vi "ABB enter winding data.vi"(9 "Efficiency Units":u16(ring) items=["METRIC", "IMPERIAL", "", "", ""], 10 "Efficiency Standard":u16(ring) items=["IEC", "NEMA"], 11 "Motor Type":u16(ring) items=["Wound Induction Motor", "Induction Motor", "Synchronous Motor", "Synchronous Generator"]) -> (3 "entered data":string[][](array[string]))   [LabVIEW 2017]
uses:
  <vilib>/Analysis/baseanly.llb/Mean (DBL).vi
  ABB global.vi
  <vilib>/Analysis/NI_AALBase.lvlib
panel:
  in  "Wound Motor Voltage Ratio":T1
  out "Winding ºC":T2 {"Avrg ºC" format="%#.3g"; "Temperature (ºC)" format="%#.2g"}
  out "Additional Temp":T3 {"Avrg cold air ºC" format="%#.3g"; "Avrg warm air ºC" format="%#.3g"; "Cold Air  (ºC)" format="%#.2g"; "Warm Air  (ºC)" format="%#.2g"}
  in  "Additional RTDs":T4={"Warm Air Ohms"=[], "Cold Air Ohms"=[], "No. Warm Air"=4, "No. Cold Air"=6} {"No. Cold Air" min=0 max=12; "No. Warm Air" min=0 max=6}
  in  "Rotor Winding Resistance":T5 {"Units" items=["Ohms", "mOhms", "uOhms"]; "Rotor K - M" format="%#.6g"; "Rotor L - M" format="%#.6g"; "Rotor K -L" format="%#.6g"}
  in  "Stator Winding resistance":T6 {"Stator U - W" format="%#.6g"; "Stator V - W" format="%#.6g"; "Units" items=["Ohms", "mOhms", "uOhms"]; "Stator U - V" format="%#.6g"}
  in  "Winding Temperatures":T7={"No. Winding ETDs"=6, "Detector Ohms"=[]} {"No. Winding ETDs" min=1 max=12}
  in  "Exit":bool
  # "Enter Winding data"
  # "20%"
  # "100%"
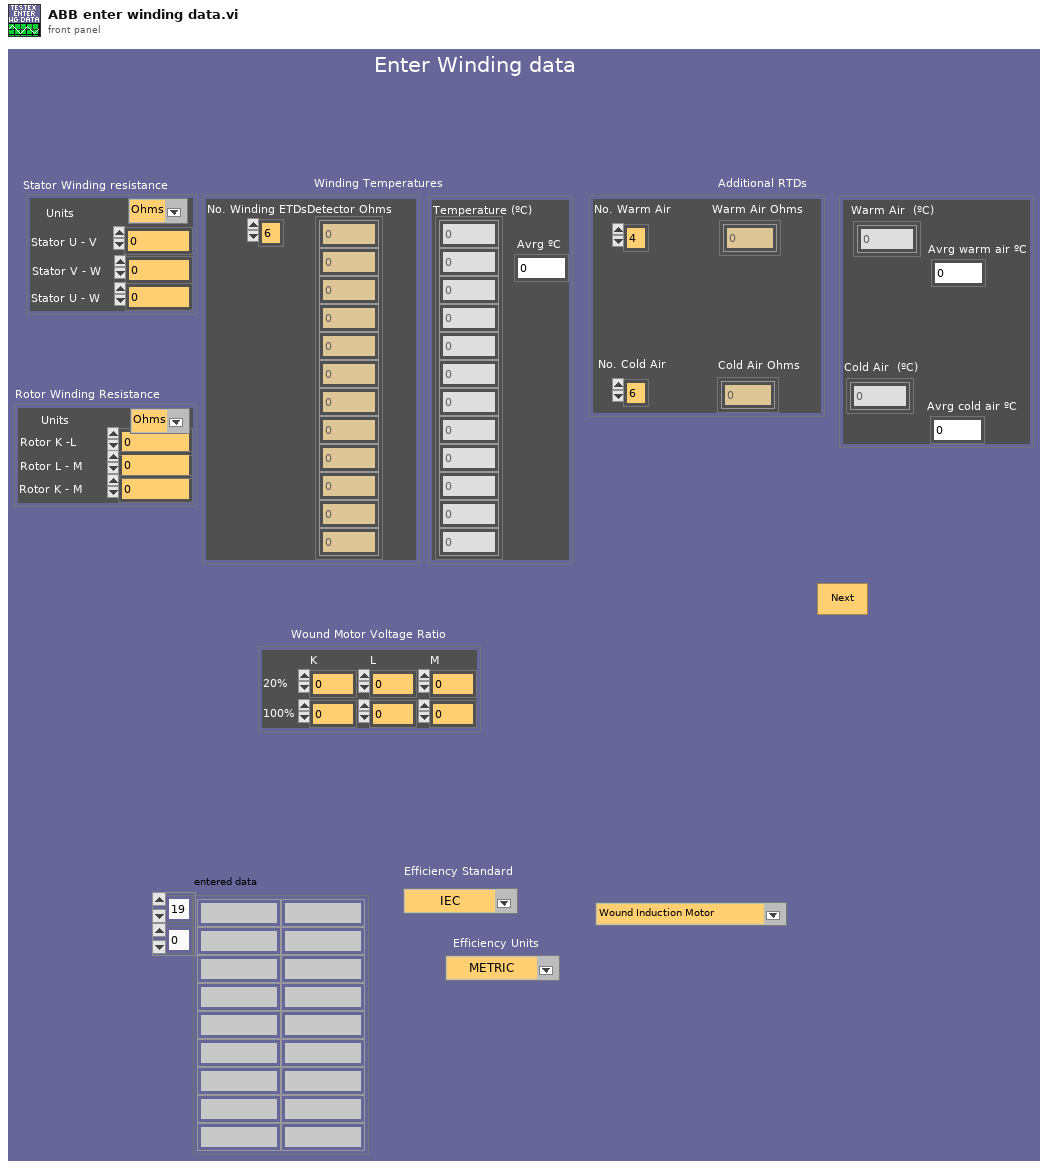
[diagram p1: front panel]
types:
  T1 = cluster{"K-20":dbl, "L-20":dbl, "M-20":dbl, "K-100":dbl, "L-100":dbl, "M-100":dbl}
  T2 = cluster{"Temperature (ºC) ":dbl[], "Avrg ºC ":dbl}
  T3 = cluster{"Warm Air  (ºC) ":dbl[], "Cold Air  (ºC) ":dbl[], "Avrg warm air ºC ":dbl, "Avrg cold air ºC":dbl}
  T4 = cluster{"Warm Air Ohms":dbl[], "Cold Air Ohms":dbl[], "No. Warm Air":i32, "No. Cold Air":i32}
  T5 = cluster{"Units":u16, "Rotor K -L":dbl, "Rotor L - M ":dbl, "Rotor K - M":dbl}
  T6 = cluster{"Units":u16, "Stator U - V":dbl, "Stator V - W":dbl, "Stator U - W":dbl}
  T7 = cluster{"No. Winding ETDs":i32, "Detector Ohms":dbl[]}
  T8 = cluster{"Selected Entries[0]":string, "Selected Entries[1]":string, "Selected Entries[2]":string, "Selected Entries[3]":string}
  T9 = cluster{"Selected Entries[0]":string, "Selected Entries[1]":string, "Selected Entries[2]":string, "Selected Entries[3]":string, "Selected Entries[4]":string}
  T10 = cluster{"Selected Entries[0]":dbl, "Selected Entries[1]":dbl, "Selected Entries[2]":dbl, "Selected Entries[3]":dbl}
  T11 = cluster{"Selected Entries[0]":dbl, "Selected Entries[1]":dbl, "Selected Entries[2]":dbl, "Selected Entries[3]":dbl, "Selected Entries[4]":dbl}
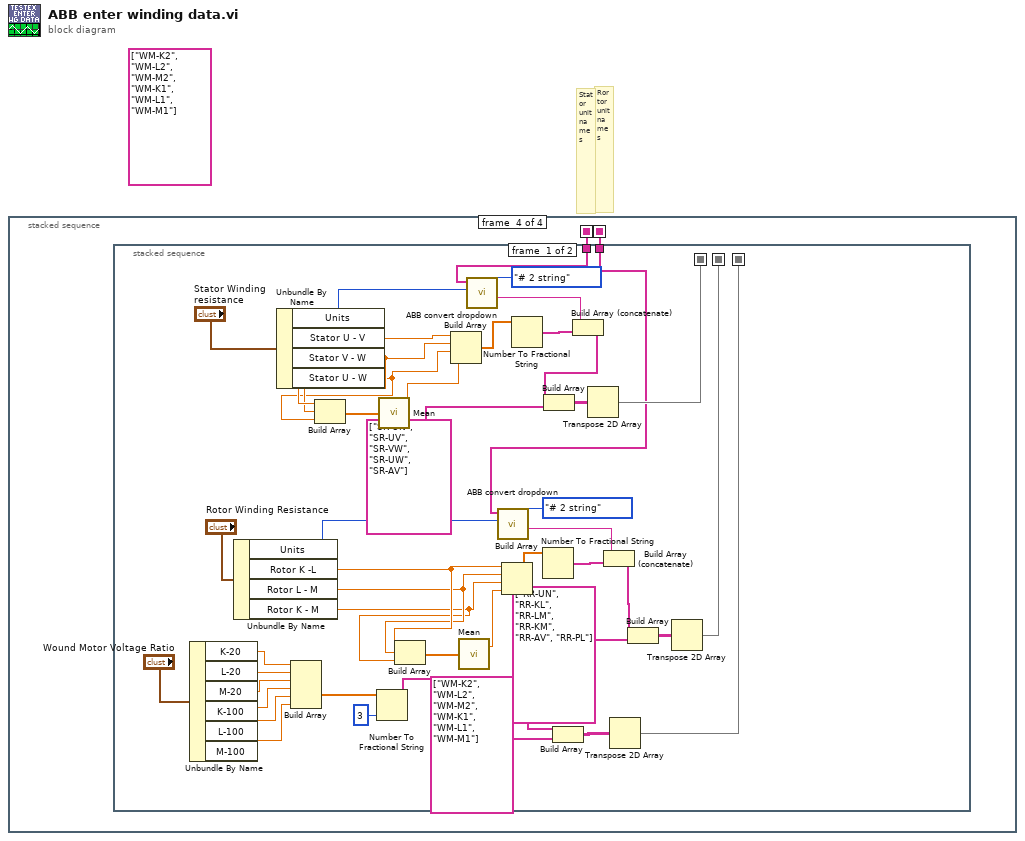
[diagram p0: block diagram]
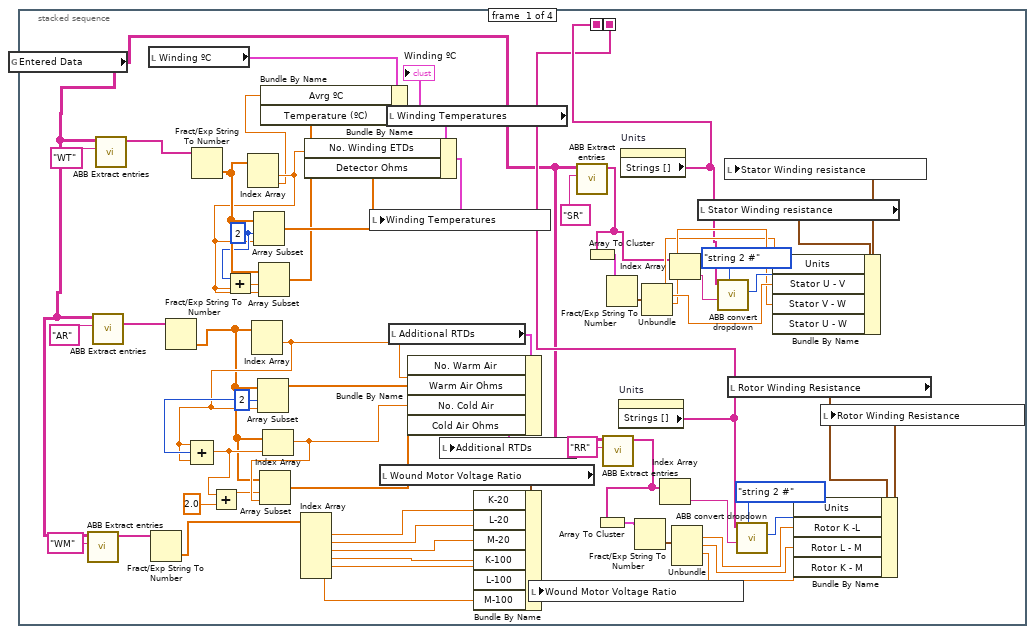
[diagram p2: hidden frame]
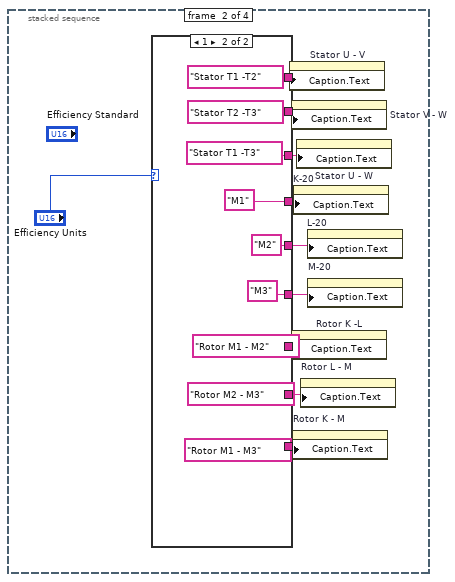
[diagram p3: hidden frame]
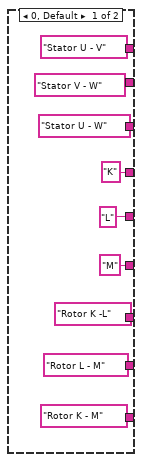
[diagram p4: hidden frame]
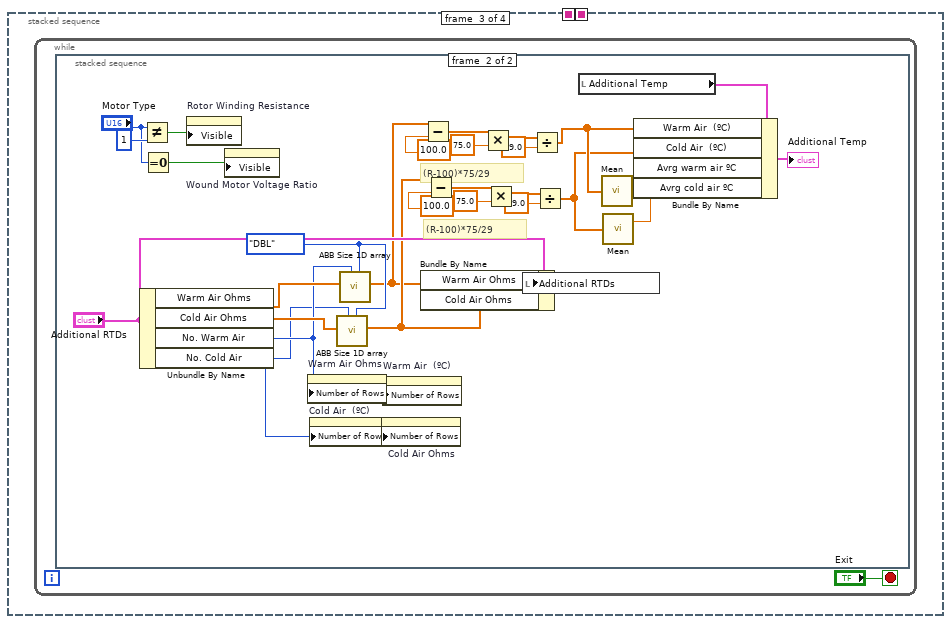
[diagram p5: hidden frame]
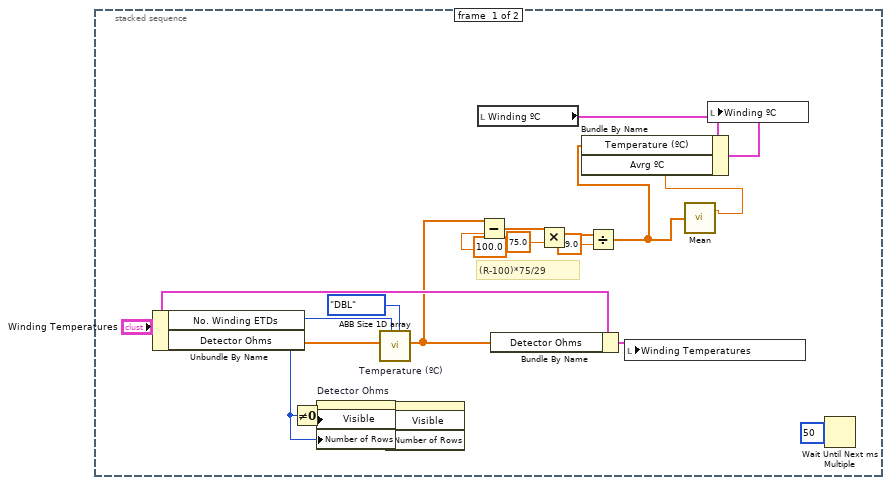
[diagram p6: hidden frame]
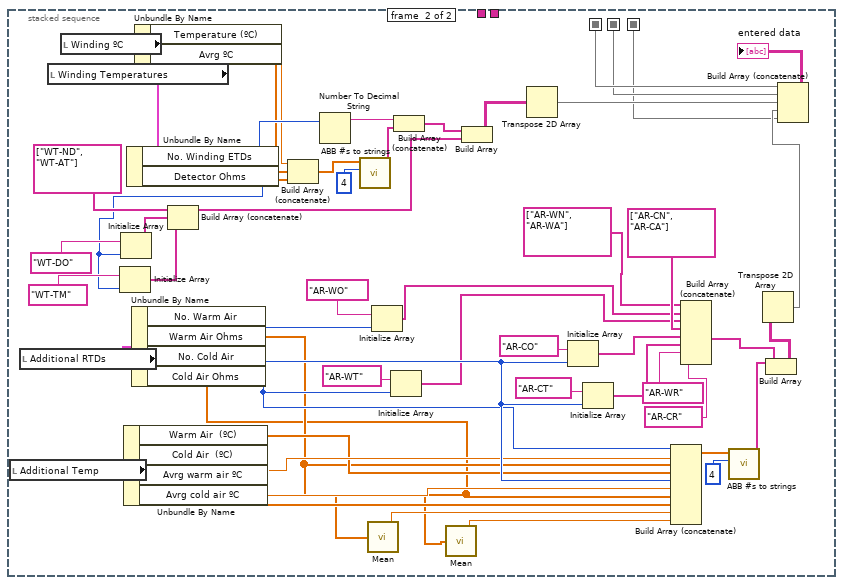
[diagram p7: hidden frame]
diagram:
  (unwired) string[] ["WM-K2", "WM-L2", "WM-M2", "WM-K1", "WM-L1", "WM-M1"]
  # "Rortor unit names"
  # "Stator unit names"
  n1 = stacked-sequence {
    seq-local: [w36 _ _ _] -> [_ _ _ w141]
    seq-local: [w35 _ _ _] -> [_ _ _ w140]
    frame #0 {
      w25 = 2 ("index")
      w32 = 2 ("index")
      n2 = global read "ABB global.vi" "Entered Data"() -> (w12:string[][])
      n3 = call "ABB Extract entries.vi"("Entry ID"="WM", "Entry table in"=w12) -> ("Selected Entries"=w10:string[])  [unwired: 9 in]
      n4 = call "ABB Extract entries.vi"("Entry ID"="AR", "Entry table in"=w12) -> ("Selected Entries"=w28:string[])  [unwired: 9 in]
      n5 = call "ABB Extract entries.vi"("Entry ID"="WT", "Entry table in"=w12) -> ("Selected Entries"=w60:string[])  [unwired: 9 in]
      n6 = local read "Winding ºC"() -> (w18:T2)
      n7 = Fract/Exp String To Number(string=w10) -> (number=w9:dbl[])  [unwired: 3 in, 1 out]
      n8 = Fract/Exp String To Number(string=w28) -> (number=w14:dbl[])  [unwired: 3 in, 1 out]
      n9 = Fract/Exp String To Number(string=w60) -> (number=w33:dbl[])  [unwired: 3 in, 1 out]
      n10 = Index Array(array=w33) -> (element #1=w31:dbl, element #2=w16:dbl)  [unwired: 2 in]
      n11 = Add(x=w32, y=w31) -> (x+y=w30:dbl)
      n12 = Index Array(array=w14) -> (element #1=w24:dbl)  [unwired: 2 in, 1 out]
      n13 = Compound Arithmetic op=ADD(w24, w25, w24) -> (w23:dbl)
      n14 = Add(x=w23, y=2.0) -> (x+y=w13:dbl)
      n15 = Array Subset(array=w33, index=w32, length=w31) -> (w62:dbl[])
      n16 = Array Subset(array=w14, index=w25, length=w24) -> (w26:dbl[])
      n17 = Array Subset(array=w33, index=w30, length=w31) -> (w15:dbl[])
      n18 = Bundle By Name(cluster=w18, "Avrg ºC"=w16, "Temperature (ºC)"=w15) -> (→"Winding ºC":T2)
      n19 = Index Array(array=w14, index=w23) -> (element=w21:dbl)
      n20 = Array Subset(array=w14, index=w13, length=w21) -> (w20:dbl[])
      n21 = Index Array(array=w9) -> (element #1=w7:dbl, element #2=w6:dbl, element #3=w5:dbl, element #4=w4:dbl, element #5=w3:dbl, element #6=w2:dbl)  [unwired: 6 in]
      n22 = local read "Wound Motor Voltage Ratio"() -> (w8:T1)
      n23 = local read "Winding Temperatures"() -> (w64:T7)
      n24 = Bundle By Name(cluster=w64, "No. Winding ETDs"=w31, "Detector Ohms"=w62) -> (w63:T7)
      n25 = local write "Winding Temperatures"(w63) -> ()
      n26 = local read "Additional RTDs"() -> (w27:T4)
      n27 = Bundle By Name(cluster=w27, "No. Warm Air"=w24, "Warm Air Ohms"=w26, "No. Cold Air"=w21, "Cold Air Ohms"=w20) -> (w19:T4)
      n28 = local write "Additional RTDs"(w19) -> ()
      n29 = Bundle By Name(cluster=w8, "K-20"=w7, "L-20"=w6, "M-20"=w5, "K-100"=w4, "L-100"=w3, "M-100"=w2) -> (w1:T1)
      n30 = local write "Wound Motor Voltage Ratio"(w1) -> ()
      n31 = call "ABB Extract entries.vi"("Entry ID"="SR", "Entry table in"=w12) -> ("Selected Entries"=w49:string[])  [unwired: 9 in]
      n32 = Array To Cluster(array=w49) -> (cluster=w50:T8)
      n33 = call "ABB Extract entries.vi"("Entry ID"="RR", "Entry table in"=w12) -> ("Selected Entries"=w38:string[])  [unwired: 9 in]
      n34 = Array To Cluster(array=w38) -> (cluster=w41:T9)
      n35 = Fract/Exp String To Number(string=w50) -> (number=w57:T10)  [unwired: 3 in, 1 out]
      n36 = property on="Units" class="Ring (strict)"() -> ("Strings []"=w35:string[])  [unwired: 2 in, 2 out]
      n37 = property on="Units" class="Ring (strict)"() -> ("Strings []"=w36:string[])  [unwired: 2 in, 2 out]
      n38 = Fract/Exp String To Number(string=w41) -> (number=w42:T11)  [unwired: 3 in, 1 out]
      n39 = Unbundle(w57) -> ("Selected Entries[1]"=w54:dbl, "Selected Entries[2]"=w53:dbl, "Selected Entries[3]"=w52:dbl)  [unwired: 1 out]
      n40 = Index Array(array=w38) -> (element=w37:string)  [unwired: 1 in]
      n41 = Index Array(array=w49) -> (element=w48:string)  [unwired: 1 in]
      n42 = Unbundle(w42) -> ("Selected Entries[1]"=w45:dbl, "Selected Entries[2]"=w46:dbl, "Selected Entries[3]"=w47:dbl)  [unwired: 2 out]
      n43 = local read "Stator Winding resistance"() -> (w59:T6)
      n44 = call "ABB convert dropdown.vi"("Mode"=enum16{"# 2 string", "string 2 #"}."string 2 #", "String in"=w48, "Strings"=w36) -> ("#out"=w56:i32)  [unwired: 7 in, 1 out]
      n45 = local read "Rotor Winding Resistance"() -> (w40:T5)
      n46 = call "ABB convert dropdown.vi"("Mode"=enum16{"# 2 string", "string 2 #"}."string 2 #", "String in"=w37, "Strings"=w35) -> ("#out"=w43:i32)  [unwired: 7 in, 1 out]
      n47 = Bundle By Name(cluster=w59, "Units"=w56, "Stator U - V"=w54, "Stator V - W"=w53, "Stator U - W"=w52) -> (w58:T6)
      n48 = local write "Stator Winding resistance"(w58) -> ()
      n49 = Bundle By Name(cluster=w40, "Units"=w43, "Rotor K -L"=w45, "Rotor L - M"=w46, "Rotor K - M"=w47) -> (w39:T5)
      n50 = local write "Rotor Winding Resistance"(w39) -> ()
    }
    frame #1 {
      n51 = case shown="1" "Efficiency Units" {
        tunnel: ["Stator U - V" ("Caption.Text") "Stator T1 -T2" ("Caption.Text")] -> w74
        tunnel: ["Stator V - W" ("Caption.Text") "Stator T2 -T3" ("Caption.Text")] -> w73
        tunnel: ["Stator U - W" ("Caption.Text") "Stator T1 -T3" ("Caption.Text")] -> w72
        tunnel: ["K" ("Caption.Text") "M1" ("Caption.Text")] -> w69
        tunnel: ["L" ("Caption.Text") "M2" ("Caption.Text")] -> w71
        tunnel: ["M" ("Caption.Text") "M3" ("Caption.Text")] -> w70
        tunnel: ["Rotor K -L" "Rotor M1 - M2"] -> w68
        tunnel: ["Rotor L - M" "Rotor M2 - M3"] -> w67
        tunnel: ["Rotor K - M" "Rotor M1 - M3"] -> w66
        frame 0, Default {
        }
        frame 1 {
        }
      }
      n52 = property on="Stator U - V" class="DigNum (strict)"("Caption.Text"=w74) -> ()  [unwired: 2 in, 2 out]
      n53 = property on="Stator V - W" class="DigNum (strict)"("Caption.Text"=w73) -> ()  [unwired: 2 in, 2 out]
      n54 = property on="Rotor K -L" class="DigNum (strict)"("Caption.Text"=w68) -> ()  [unwired: 2 in, 2 out]
      n55 = property on="Rotor K - M" class="DigNum (strict)"("Caption.Text"=w66) -> ()  [unwired: 2 in, 2 out]
      n56 = property on="K-20" class="DigNum (strict)"("Caption.Text"=w69) -> ()  [unwired: 2 in, 2 out]
      n57 = property on="Stator U - W" class="DigNum (strict)"("Caption.Text"=w72) -> ()  [unwired: 2 in, 2 out]
      n58 = property on="Rotor L - M" class="DigNum (strict)"("Caption.Text"=w67) -> ()  [unwired: 2 in, 2 out]
      n59 = property on="L-20" class="DigNum (strict)"("Caption.Text"=w71) -> ()  [unwired: 2 in, 2 out]
      n60 = property on="M-20" class="DigNum (strict)"("Caption.Text"=w70) -> ()  [unwired: 2 in, 2 out]
    }
    frame #2 {
      n61 = while {
        stop <- "Exit" stop-if-true
        n62 = stacked-sequence {
          frame #0 {
            # "(R-100)*75/29"
            n63 = Unbundle By Name("Winding Temperatures") -> ("No. Winding ETDs"=w104:i32, "Detector Ohms"=w108:dbl[])
            n64 = Not Equal To 0?(x=w104) -> (x != 0?=w105:bool)
            n65 = property on="Detector Ohms" class="Arr (strict)"("Visible"=w105, "Number of Rows"=w104) -> ()  [unwired: 2 in, 2 out]
            n66 = call "ABB Size 1D array.vi"("Type"=enum16{"Integer", "DBL", "STRING", "BOOLEAN"}."DBL", "Size"=w104, "DBL Array In"=w108) -> ("DBL Array out"=w99:dbl[])  [unwired: 5 in, 3 out]
            n67 = property on="Temperature (ºC)" class="Arr (strict)"("Visible"=w105, "Number of Rows"=w104) -> ()  [unwired: 2 in, 2 out]
            n68 = local read "Winding ºC"() -> (w97:T2)
            n69 = Subtract(x=w99, y=100.0) -> (x-y=w100:dbl[])
            n70 = Bundle By Name(cluster="Winding Temperatures", "Detector Ohms"=w99) -> (w106:T7)
            n71 = Multiply(x=w100, y=75.0) -> (x*y=w102:dbl[])
            n72 = Divide(x=w102, y=29.0) -> (x/y=w94:dbl[])
            n73 = local write "Winding Temperatures"(w106) -> ()
            n74 = call-poly <vilib>:"Mean.vi"("X"=w94) -> ("mean"=w95:dbl)  [unwired: 1 out]
            n75 = Bundle By Name(cluster=w97, "Temperature (ºC)"=w94, "Avrg ºC"=w95) -> (w96:T2)
            n76 = local write "Winding ºC"(w96) -> ()
            n77 = Wait Until Next ms Multiple(millisecond multiple=u32 50) -> ()  [unwired: 1 out]
          }
          frame #1 {
            w135 = enum16{"Integer", "DBL", "STRING", "BOOLEAN"}."DBL" ("Type")
            # "(R-100)*75/29"
            # "(R-100)*75/29"
            n78 = Unbundle By Name("Additional RTDs") -> ("Warm Air Ohms"=w139:dbl[], "Cold Air Ohms"=w138:dbl[], "No. Warm Air"=w137:i32, "No. Cold Air"=w136:i32)
            n79 = Not Equal?(x="Motor Type", y=u16 1) -> (x != y?=w113:bool)
            n80 = Equal To 0?(x="Motor Type") -> (x = 0?=w111:bool)
            n81 = property on="Rotor Winding Resistance" class="Clust (strict)"("Visible"=w113) -> ()  [unwired: 2 in, 2 out]
            n82 = property on="Wound Motor Voltage Ratio" class="Clust (strict)"("Visible"=w111) -> ()  [unwired: 2 in, 2 out]
            n83 = property on="Warm Air Ohms" class="Arr (strict)"("Number of Rows"=w137) -> ()  [unwired: 2 in, 2 out]
            n84 = property on="Cold Air  (ºC)" class="Arr (strict)"("Number of Rows"=w136) -> ()  [unwired: 2 in, 2 out]
            n85 = call "ABB Size 1D array.vi"("Type"=w135, "Size"=w136, "DBL Array In"=w138) -> ("DBL Array out"=w122:dbl[])  [unwired: 5 in, 3 out]
            n86 = call "ABB Size 1D array.vi"("Type"=w135, "Size"=w137, "DBL Array In"=w139) -> ("DBL Array out"=w121:dbl[])  [unwired: 5 in, 3 out]
            n87 = property on="Cold Air Ohms" class="Arr (strict)"("Number of Rows"=w136) -> ()  [unwired: 2 in, 2 out]
            n88 = property on="Warm Air  (ºC)" class="Arr (strict)"("Number of Rows"=w137) -> ()  [unwired: 2 in, 2 out]
            n89 = Bundle By Name(cluster="Additional RTDs", "Warm Air Ohms"=w121, "Cold Air Ohms"=w122) -> (w133:T4)
            n90 = Subtract(x=w121, y=100.0) -> (x-y=w129:dbl[])
            n91 = Subtract(x=w122, y=100.0) -> (x-y=w126:dbl[])
            n92 = Multiply(x=w129, y=75.0) -> (x*y=w131:dbl[])
            n93 = Multiply(x=w126, y=75.0) -> (x*y=w124:dbl[])
            n94 = local write "Additional RTDs"(w133) -> ()
            n95 = Divide(x=w131, y=29.0) -> (x/y=w118:dbl[])
            n96 = Divide(x=w124, y=29.0) -> (x/y=w117:dbl[])
            n97 = local read "Additional Temp"() -> (w120:T3)
            n98 = call-poly <vilib>:"Mean.vi"("X"=w118) -> ("mean"=w116:dbl)  [unwired: 1 out]
            n99 = call-poly <vilib>:"Mean.vi"("X"=w117) -> ("mean"=w115:dbl)  [unwired: 1 out]
            n100 = Bundle By Name(cluster=w120, "Warm Air  (ºC)"=w118, "Cold Air  (ºC)"=w117, "Avrg warm air ºC"=w116, "Avrg cold air ºC"=w115) -> (→"Additional Temp":T3)
          }
        }
      }
    }
    frame #3 {
      n101 = stacked-sequence {
        seq-local: [w168 _] -> [_ w228]
        seq-local: [w167 _] -> [_ w227]
        seq-local: [w143 _] -> [_ w187]
        tunnel: w141 -> [w166 _]
        tunnel: w140 -> [w165 _]
        frame #0 {
          n102 = Unbundle By Name("Wound Motor Voltage Ratio") -> ("K-20"=w153:dbl, "L-20"=w152:dbl, "M-20"=w151:dbl, "K-100"=w150:dbl, "L-100"=w149:dbl, "M-100"=w148:dbl)
          n103 = Unbundle By Name("Rotor Winding Resistance") -> ("Units"=w184:u16, "Rotor K -L"=w157:dbl, "Rotor L - M"=w156:dbl, "Rotor K - M"=w155:dbl)
          n104 = Unbundle By Name("Stator Winding resistance") -> ("Units"=w175:u16, "Stator U - V"=w164:dbl, "Stator V - W"=w163:dbl, "Stator U - W"=w162:dbl)
          n105 = Build Array(w153, w152, w151, w150, w149, w148) -> (w147:dbl[])
          n106 = Build Array(w164, w163, w162) -> (w161:dbl[])
          n107 = Number To Fractional String(number=w147, precision (6)=i16 3) -> (F-format string=w145:string[])  [unwired: 2 in]
          n108 = call-poly <vilib>:"Mean.vi"("X"=w161) -> ("mean"=w160:dbl)  [unwired: 1 out]
          n109 = Build Array(w157, w156, w155) -> (w159:dbl[])
          n110 = Build Array(w164, w163, w162, w160) -> (w173:dbl[])
          n111 = call-poly <vilib>:"Mean.vi"("X"=w159) -> ("mean"=w158:dbl)  [unwired: 1 out]
          n112 = call "ABB convert dropdown.vi"("Mode"=enum16{"# 2 string", "string 2 #"}."# 2 string", "# in"=w175, "Strings"=w166) -> ("String out"=w177:string)  [unwired: 7 in, 1 out]
          n113 = call "ABB convert dropdown.vi"("Mode"=enum16{"# 2 string", "string 2 #"}."# 2 string", "# in"=w184, "Strings"=w165) -> ("String out"=w186:string)  [unwired: 7 in, 1 out]
          n114 = Build Array(w157, w156, w155, w158) -> (w182:dbl[])
          n115 = Number To Fractional String(number=w173) -> (F-format string=w174:string[])  [unwired: 3 in]
          n116 = Number To Fractional String(number=w182) -> (F-format string=w183:string[])  [unwired: 3 in]
          n117 = Build Array(w145, string[] ["WM-K2", "WM-L2", "WM-M2", "WM-K1", "WM-L1", "WM-M1"]) -> (w144:string[][])
          n118 = Build Array (concatenate)(w177, w174) -> (w172:string[])
          n119 = Build Array(w172, string[] ["SR-UN", "SR-UV", "SR-VW", "SR-UW", "SR-AV"]) -> (w170:string[][])
          n120 = Transpose 2D Array(2D array=w170) -> (transposed array=w168:string[][])
          n121 = Build Array (concatenate)(w186, w183) -> (w181:string[])
          n122 = Transpose 2D Array(2D array=w144) -> (transposed array=w143:string[][])
          n123 = Build Array(w181, string[] ["RR-UN", "RR-KL", "RR-LM", "RR-KM", "RR-AV", "RR-PL"]) -> (w179:string[][])
          n124 = Transpose 2D Array(2D array=w179) -> (transposed array=w167:string[][])
        }
        frame #1 {
          n125 = local read "Additional Temp"() -> (w219:T3)
          n126 = local read "Additional RTDs"() -> (w220:T4)
          n127 = local read "Winding Temperatures"() -> (w239:T7)
          n128 = local read "Winding ºC"() -> (w196:T2)
          n129 = Unbundle By Name(w219) -> ("Warm Air  (ºC)"=w205:dbl[], "Cold Air  (ºC)"=w209:dbl[], "Avrg warm air ºC"=w206:dbl, "Avrg cold air ºC"=w210:dbl)
          n130 = Unbundle By Name(w239) -> ("No. Winding ETDs"=w223:i32, "Detector Ohms"=w238:dbl[])
          n131 = Initialize Array("WT-TM", w223) -> (w225:string[])
          n132 = Initialize Array("WT-DO", w223) -> (w234:string[])
          n133 = Unbundle By Name(w220) -> ("No. Warm Air"=w207:i32, "Warm Air Ohms"=w193:dbl[], "No. Cold Air"=w211:i32, "Cold Air Ohms"=w190:dbl[])
          n134 = Unbundle By Name(w196) -> ("Temperature (ºC)"=w194:dbl[], "Avrg ºC"=w195:dbl)
          n135 = Build Array (concatenate)(string[] ["WT-ND", "WT-AT"], w234, w225) -> (w231:string[])
          n136 = Build Array (concatenate)(w195, w238, w194) -> (w237:dbl[])
          n137 = Number To Decimal String(number=w223) -> (decimal integer string=w221:string)  [unwired: 1 in]
          n138 = call "ABB #s to strings.vi"("Precision"=i16 4 ("precision (6)"), "Numbers in"=w237) -> ("Strings out"=w232:string[])  [unwired: 9 in]
          n139 = call-poly <vilib>:"Mean.vi"("X"=w193) -> ("mean"=w192:dbl)  [unwired: 1 out]
          n140 = Initialize Array("AR-WO", w207) -> (w202:string[])
          n141 = Initialize Array("AR-WT", w207) -> (w201:string[])
          n142 = Build Array (concatenate)(w221, w232) -> (w222:string[])
          n143 = call-poly <vilib>:"Mean.vi"("X"=w190) -> ("mean"=w191:dbl)  [unwired: 1 out]
          n144 = Build Array(w222, w231) -> (w233:string[][])
          n145 = Transpose 2D Array(2D array=w233) -> (transposed array=w230:string[][])
          n146 = Initialize Array("AR-CO", w211) -> (w214:string[])
          n147 = Initialize Array("AR-CT", w211) -> (w216:string[])
          n148 = Build Array (concatenate)(w207, w206, w193, w205, w211, w210, w190, w209, w192, w191) -> (w204:dbl[])
          n149 = Build Array (concatenate)(string[] ["AR-WN", "AR-WA"], w202, w201, string[] ["AR-CN", "AR-CA"], w214, w216, "AR-WR", "AR-CR") -> (w197:string[])
          n150 = call "ABB #s to strings.vi"("Precision"=i16 4 ("precision (6)"), "Numbers in"=w204) -> ("Strings out"=w198:string[])  [unwired: 9 in]
          n151 = Build Array(w198, w197) -> (w200:string[][])
          n152 = Transpose 2D Array(2D array=w200) -> (transposed array=w199:string[][])
          n153 = Build Array (concatenate)(w228, w227, w230, w199, w187) -> (→"entered data":string[][])
        }
      }
    }
  }
